vi "Example Trigger Event.vi"() -> ()   [LabVIEW 2015]
uses:
  Event Input/Event Input.lvclass/Event Input.ctl
  Result/result.lvclass
  input/input.lvclass
  Event Input/Event Input.lvclass
panel:
  out "Connected":bool
  in  "Trigger Button":bool
  in  "Stop Button":bool
  out "Error Out":errorcluster
  out "Answer":string
  in  "Greeting":string="Greetings from LabView"
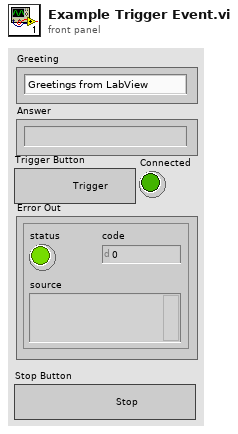
[diagram p1: front panel]
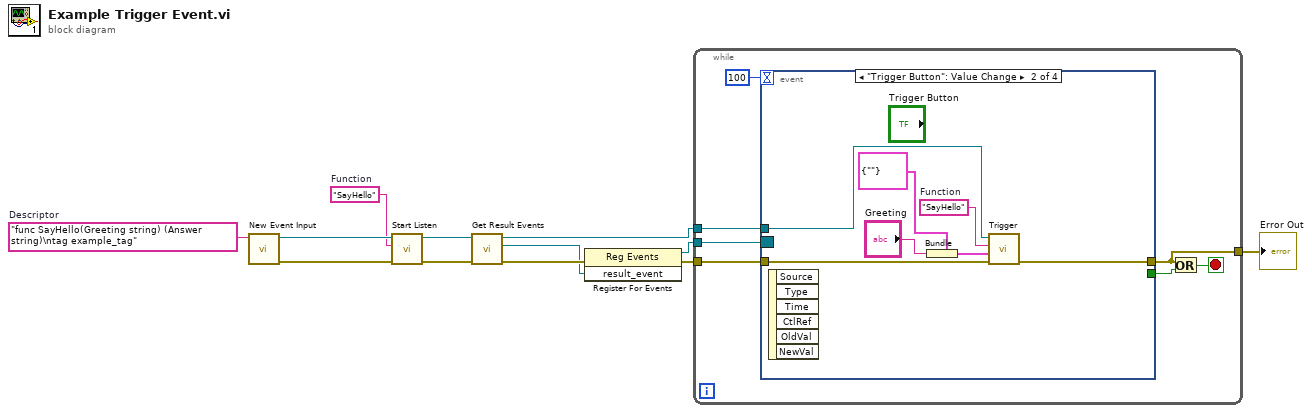
[diagram p0: block diagram]
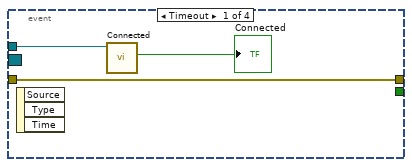
[diagram p2: hidden frame]
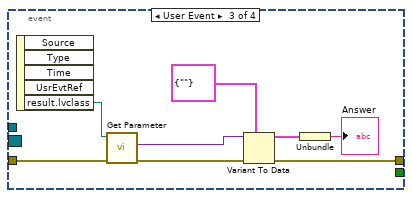
[diagram p3: hidden frame]
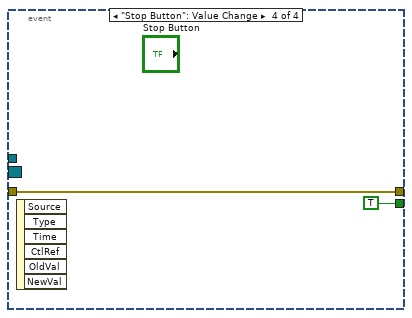
[diagram p4: hidden frame]
diagram:
  w12 = "func SayHello(Greeting string) (Answer string)\ntag example_tag"  # Descriptor
  w9 = "SayHello"  # Function
  n1 = call "New Event Input.vi"("Descriptor"=w12) -> ("error out"=w10:errorcluster, "event_input out"=w11:refnum<class "Event Input.lvclass">)  [unwired: 9 in]
  n2 = call "Start Listen.vi"("error in (no error)"=w10, "Function"=w9, "input in"=w11) -> ("error out"=w7:errorcluster, "input out"=w8:refnum<class "Event Input.lvclass">)  [unwired: 7 in]
  n3 = call "Get Result Events.vi"("error in (no error)"=w7, "event_input in"=w8) -> ("error out"=w6:errorcluster, "result_event"=w5:refnum<user-event>, "event_input out"=w3:refnum<class "Event Input.lvclass">)  [unwired: 7 in]
  n4 = register-events(error in=w6, w5) -> (reference out=w4:refnum<event-registration>, error out=w2:errorcluster)  [unwired: 1 in]
  n5 = while {
    tunnel: w4 -> [w19]
    tunnel: w3 -> [w17]
    tunnel: w2 -> [w16]
    tunnel: [w15] -> w1
    stop <- w13 stop-if-true
    n6 = event shown="[1] \"Trigger Button\": Value Change" {
      selector: w19 -> [_ _ _ _]
      dyn-events: _ -> [_ _ _ _]
      timeout: 100 -> [_ _ _ _]
      tunnel: w17 -> [w21 w25 _ _]
      tunnel: w16 -> [w20 w24 w31 w38]
      tunnel: [w20 w23 w30 w38] -> w15
      tunnel: [_ _ _ TRUE ("Stop Button")] -> w14
      event Timeout {
        n7 = event-data() -> ()  [unwired: 1 in, 3 out]
        n8 = call "Connected.vi"("input in"=w21) -> ("connected"=→"Connected":bool)  [unwired: 8 in, 2 out]
      }
      event "Trigger Button": Value Change {
        w26 = "SayHello"  # Function
        n9 = event-data() -> ()  [unwired: 1 in, 6 out]
        n10 = Bundle(cluster=cluster{"Greeting":string} {"Greeting"=""}, "Greeting"="Greeting") -> (w29:cluster{"Greeting":string})
        n11 = call "Trigger.vi"("error in (no error)"=w24, "Parameter"=w29, "Function"=w26, "input in"=w25) -> ("error out"=w23:errorcluster)  [unwired: 6 in, 1 out]
      }
      event User Event {
        n12 = event-data() -> ("result.lvclass"=w32:refnum<class "result.lvclass">)  [unwired: 1 in, 4 out]
        n13 = call-dynamic "Get Parameter.vi"("error in (no error)"=w31, "result in"=w32) -> ("error out"=w37:errorcluster, "Data"=w36:variant)  [unwired: 7 in, 1 out]
        n14 = Variant To Data(error in=w37, type=cluster{"Answer":string} {"Answer"=""}, Variant=w36) -> (data=w34:cluster{"Answer":string}, error out=w30:errorcluster)
        n15 = Unbundle(w34) -> ("Answer"=→"Answer":string)
      }
      event "Stop Button": Value Change {
        n16 = event-data() -> ()  [unwired: 1 in, 6 out]
      }
    }
    n17 = Or(x=w15, y=w14) -> (x .or. y?=w13:bool)
  }
  "Error Out" <- w1
